vi "close.vi"(8 "error in":errorcluster, 11 "Array of Controller Status":T1) -> (0 "error out":errorcluster)   [LabVIEW 2013, in "PI_Piezo.lvclass"]
uses:
  PI_Piezo.lvclass
  status.ctl
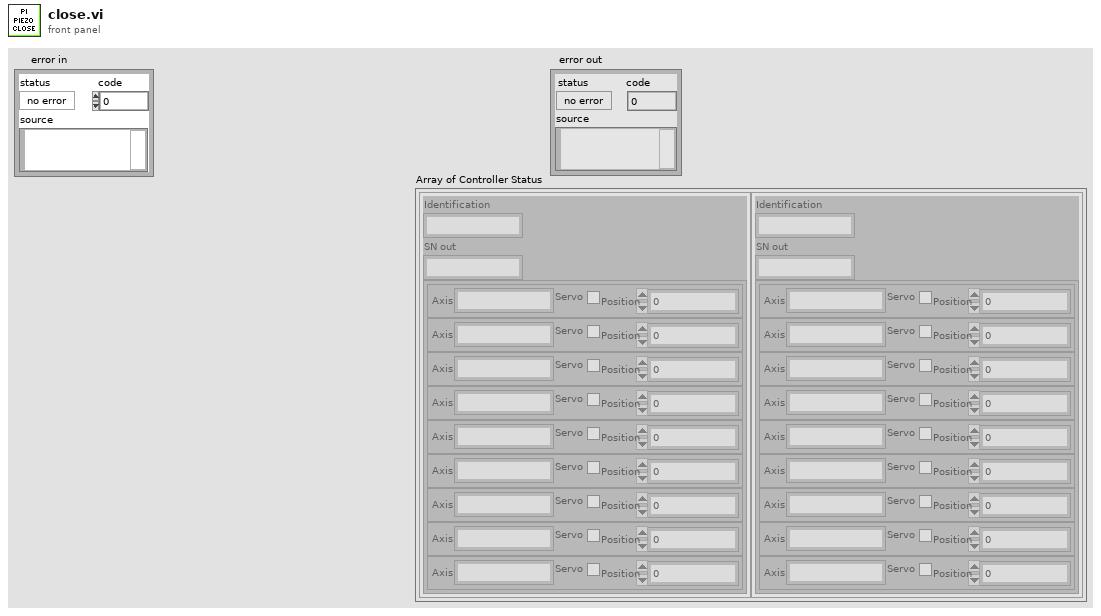
[diagram p1: front panel]
types:
  T1 = typedef "PI_Piezo.lvclass/status.ctl" = cluster{"Identification":string, "SN out":string, cluster{"Axis":string, "Servo":bool, "Position":dbl}[]}[]
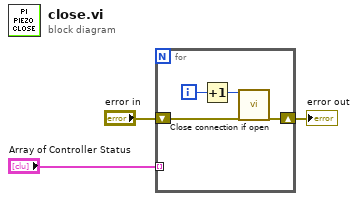
[diagram p0: block diagram]
diagram:
  n1 = for {
    shift-right: [w6] -> w2
    shift-left: "error in" -> [w7]
    tunnel: "Array of Controller Status" -> [_] mode=indexing
    i -> [w5]
    n2 = Increment(x=w5) -> (x+1=w4:i32)
    n3 = call "Close connection if open.vi"("System no."=w4, "error in"=w7) -> ("error out"=w6:errorcluster)  [unwired: 16 in, 1 out]
  }
  "error out" <- w2
